vi "Write ConfigInterface.vi"(10 "ConfigInterface":refnum<class "ConfigInterface.lvclass">, 11 "GUI in":refnum<class "GUI.lvclass">) -> (3 "GUI out":refnum<class "GUI.lvclass">)   [LabVIEW 2019, in "GUI.lvclass"]
uses:
  GUI.lvclass
  ConfigInterface_class/ConfigInterface.lvclass
  GUI.lvclass/GUI.ctl
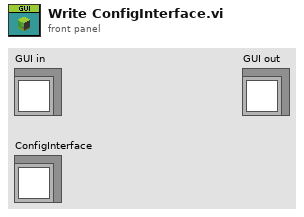
[diagram p1: front panel]
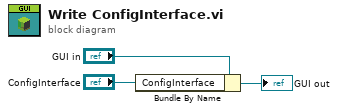
[diagram p0: block diagram]
diagram:
  n1 = Bundle By Name(cluster="GUI in", "ConfigInterface"="ConfigInterface") -> (→"GUI out":refnum<class "GUI.lvclass">)
